vi "Read Symbol Information.vi"(8 "error in (no error)":errorcluster, 10 "Name":string, 11 "TwinCAT ADS in":refnum<class "TwinCAT ADS.lvclass">) -> (0 "error out":errorcluster, 1 "Symbol Information":T1 {"Type ID" items=["ADST_VOID"=0, "ADST_INT16"=2, "ADST_INT32"=3, "ADST_REAL32"=4, "ADST_REAL64"=5, "ADST_INT8"=16, "ADST_UINT8"=17, "ADST_UINT16"=18, "ADST_UINT32"=19, "ADST_INT64"=20, "ADST_UINT64"=21, "ADST_STRING"=30, "ADST_WSTRING"=31, "ADST_REAL80"=32, "ADST_BIT"=33, "ADST_MAXTYPES"=34, "ADST_BIGTYPE"=65]; "Type Category" items=["Unknown, None"=0, "Primitive"=1, "Alias"=2, "Enum"=3, "Array"=4, "Struct"=5, "FunctionBlock"=6, "Program"=7, "Function"=8, "SubRange"=9, "String"=10, "Bitset"=12, "Pointer"=13, "Union"=14, "Reference"=15, "Interface"=16]}, 3 "TwinCAT ADS out":refnum<class "TwinCAT ADS.lvclass">)   [LabVIEW 2018, in "TwinCAT ADS.lvclass"]
uses:
  TwinCAT ADS.lvclass
  Controls/Symbol Information.ctl
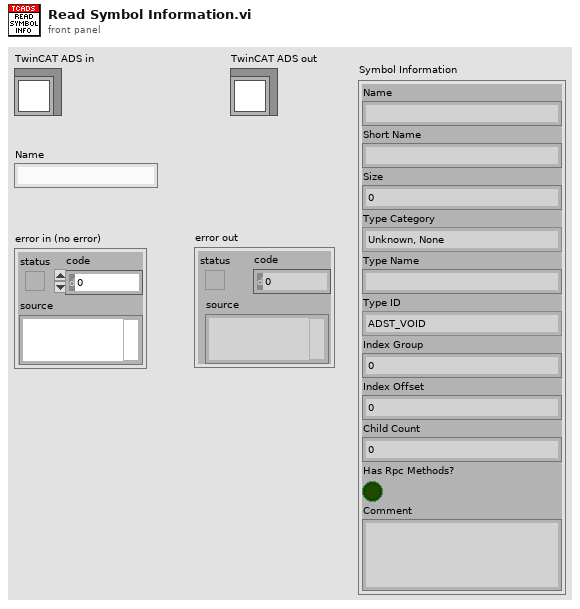
[diagram p1: front panel]
types:
  T1 = typedef "TwinCAT ADS.lvclass/Symbol Information.ctl" = cluster{"Name":string, "Short Name":string, "Size":i32, "Type Category":i32, "Type Name":string, "Type ID":i32, "Index Group":i64, "Index Offset":i64, "Child Count":i32, "Has Rpc Methods?":bool, "Comment":string}
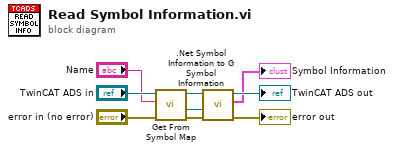
[diagram p0: block diagram]
diagram:
  n1 = call "Get From Symbol Map.vi"("error in (no error)"="error in (no error)", "Symbol Name"="Name", "TwinCAT ADS in"="TwinCAT ADS in") -> ("error out"=w4:errorcluster, ".NET Symbol Information"=w2:refnum<k24>, "TwinCAT ADS out"=w3:refnum<class "TwinCAT ADS.lvclass">)  [unwired: 6 in]
  n2 = call ".Net Symbol Information to G Symbol Information.vi"("TwinCAT ADS in"=w3, ".NET AdsSymbolInfo"=w2, "error in (no error)"=w4) -> ("TwinCAT ADS out"=→"TwinCAT ADS out":refnum<class "TwinCAT ADS.lvclass">, "Symbol Information"=→"Symbol Information":T1, "error out"=→"error out":errorcluster)  [unwired: 5 in]
